vi "WriteRebootDebugLog.vi"(7 "operation (0:open)":T1(ring)=enum."replace or create", 8 "error in":errorcluster, 11 "session":refnum<k21>) -> (0 "error out":errorcluster)   [LabVIEW 2017, in "SystemInfoProcess.lvlib"]
uses:
  <vilib>/addons/SystemInfoProcess/SystemInfoProcess.lvlib
  <vilib>/addons/InsightCM/Devices/Shared/Common/Controller/Controller.lvlib
  <vilib>/addons/InsightCM/Utilities/GlobalConfiguration/GlobalConfiguration.lvlib
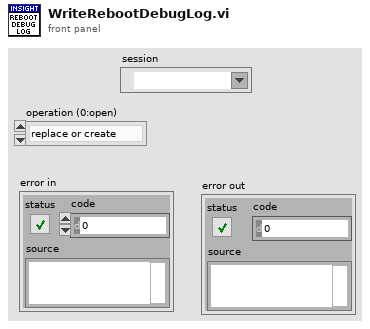
[diagram p1: front panel]
types:
  T1 = enum16{"open", "replace", "create", "open or create", "replace or create", "replace or create with confirmation"}
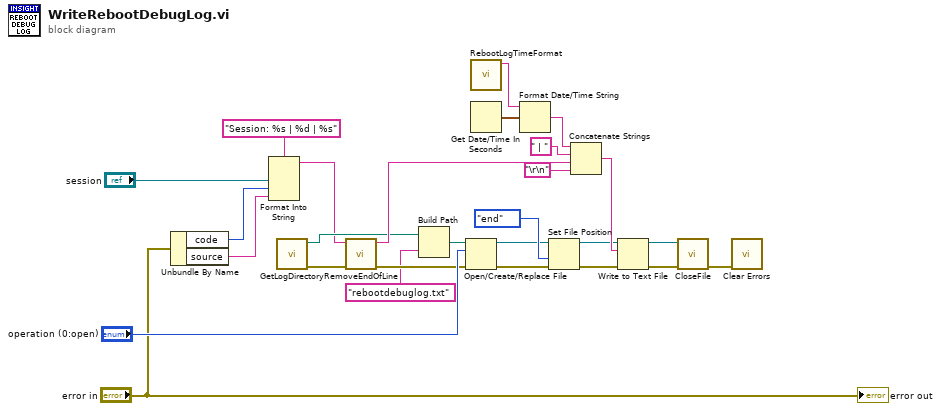
[diagram p0: block diagram]
diagram:
  n1 = Unbundle By Name("error in") -> ("code"=w3:i32, "source"=w2:string)
  n2 = Format Into String(format string="Session: %s | %d | %s", "session", w3, w2) -> (resulting string=w1:string)  [unwired: 2 in, 1 out]
  n3 = call <vilib>:"GetLogDirectory.vi"() -> ("error out"=w6:errorcluster, "log dir"=w7:path)  [unwired: 10 in]
  n4 = call <vilib>:"RemoveEndOfLine.vi"("error in"=w6, "reboot log text"=w1) -> ("error out"=w14:errorcluster, "reboot log text out"=w13:string)  [unwired: 8 in]
  n5 = Build Path(base path=w7, name or relative path="rebootdebuglog.txt") -> (appended path=w18:path)
  n6 = Open/Create/Replace File(file path (use dialog)=w18, error in=w14, operation (0:open)="operation (0:open)") -> (refnum out=w20:refnum<file>, error out=w22:errorcluster)  [unwired: 3 in, 1 out]
  n7 = call <vilib>:"RebootLogTimeFormat.vi"() -> ("time format"=w15:string)  [unwired: 11 in]
  n8 = Get Date/Time In Seconds() -> (seconds since 1Jan1904=w27:timestamp)
  n9 = Format Date/Time String(time format string (%c)=w15, seconds (now)=w27) -> (date/time string=w26:string)  [unwired: 1 in]
  n10 = Set File Position(refnum=w20, from (0:start)=enum16{"start", "end", "current"}."end", error in=w22) -> (refnum out=w23:refnum<file>, error out=w24:errorcluster)  [unwired: 1 in]
  n11 = Concatenate Strings(w26, " | " ("string"), w13, "\r\n") -> (w25:string)
  n12 = Write to Text File(file (use dialog)=w23, text=w25, error in=w24) -> (refnum out=w12:refnum<file>, error out=w11:errorcluster)  [unwired: 1 in, 1 out]
  n13 = call <vilib>:"CloseFile.vi"("error in (no error)"=w11, "file reference"=w12) -> ("error out"=w8:errorcluster)  [unwired: 9 in]
  n14 = call <vilib>:"Clear Errors.vi"("error in (no error)"=w8) -> ()  [unwired: 5 in, 2 out]
  "error out" <- "error in"
